vi "Control Panel.vi"(8 "error in (no error)":errorcluster, 11 "Lockin SR830.lvclass":refnum<class "Lockin SR830.lvclass">) -> (0 "error out":errorcluster, 3 "Lockin SR830.lvclass out":refnum<class "Lockin SR830.lvclass">)   [LabVIEW 2009, in "Lockin SR830.lvclass"]
uses:
  Lockin SR830.lvclass
  sr830/SR830.lvlib
  Main/Global/Misc.vi
  Main/Global/Flags.vi
  Global/GPIB Numbers.vi
  Utility Classes/Readable/Readable.lvclass
panel:
  out "ext?OUT":bool
  in  "ext?":bool caption="External Lock"
  in  "ch2form":T1(ring)
  in  "readcontrol":bool
  in  "ch1form":enum16{"X", "R", "X Noise", "Aux 1", "Aux 2"}(ring)
  in  "reset":bool
  out "frequnit":string
  out "freq":dbl caption="Ref Freq"
  out "ch2format":string
  out "ch1format":string
  out "ch2disp":string caption="Channel 2"
  out "ch1disp":string caption="Channel 1"
  in  "readtime":dbl=500.0 caption="Read Time (ms)"
  in  "activeread":bool caption="Auto-read?"
  in  "autophase":bool
  out "phasedisp":dbl caption="Phase"
  out "on":bool caption="Connected"
  out "sensdisp":T2(ring) caption="Sensitivity"
  out "tcdisp":T3(ring) caption="Time Const."
  in  "sens":T2(ring) caption="Sensitivity"
  in  "tc":T3(ring) caption="Time Const."
  in  "connect":bool
  in  "set":bool
  in  "read":bool
  out "active":bool caption="Active"
  in  "endprgm":bool
  # "Lock-in Detector Front Panel"
  # "**Auto-read is just for the output data."
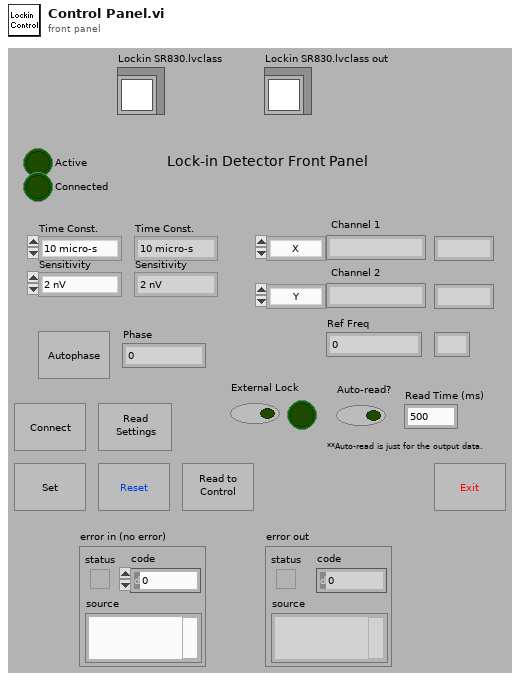
[diagram p1: front panel]
types:
  T1 = enum16{"Y", "Theta", "Y Noise", "Aux 3", "Aux 4"}
  T2 = enum16{"2 nV", "5 nV", "10 nV", "20 nV", "50 nV", "100 nV", "200 nV", "500 nV", "1 microV", "2 microV", "5 microV", "10 microV", "20 microV", "50  microV", "100  microV", "200  microV", "500  microV", "1 mV", "2 mV", "5 mV", "10 mV", "20 mV", "50 mV", "100 mV", "200  mV", "500 mV", "1 V"}
  T3 = enum16{"10 micro-s", "30 micro-s", "100 micro-s", "300 micro-s", "1 ms", "3 ms", "10 ms", "30 ms", "100 ms", "300 ms", "1 s", "3 s", "10 s", "30 s", "100 s", "300 s", "1000 s", "30000 s", "10 ks", "30 ks"}
  T4 = cluster{"name":string, "value":dbl, "unit":string}[]
  T5 = typedef "GPIB Type Def.ctl" = cluster{"Name":string, "bus":dbl, "GPIB":dbl, "GPIB as string":string, "byte":i32, "VISA Resource Name":refnum<visa-resource-name>}
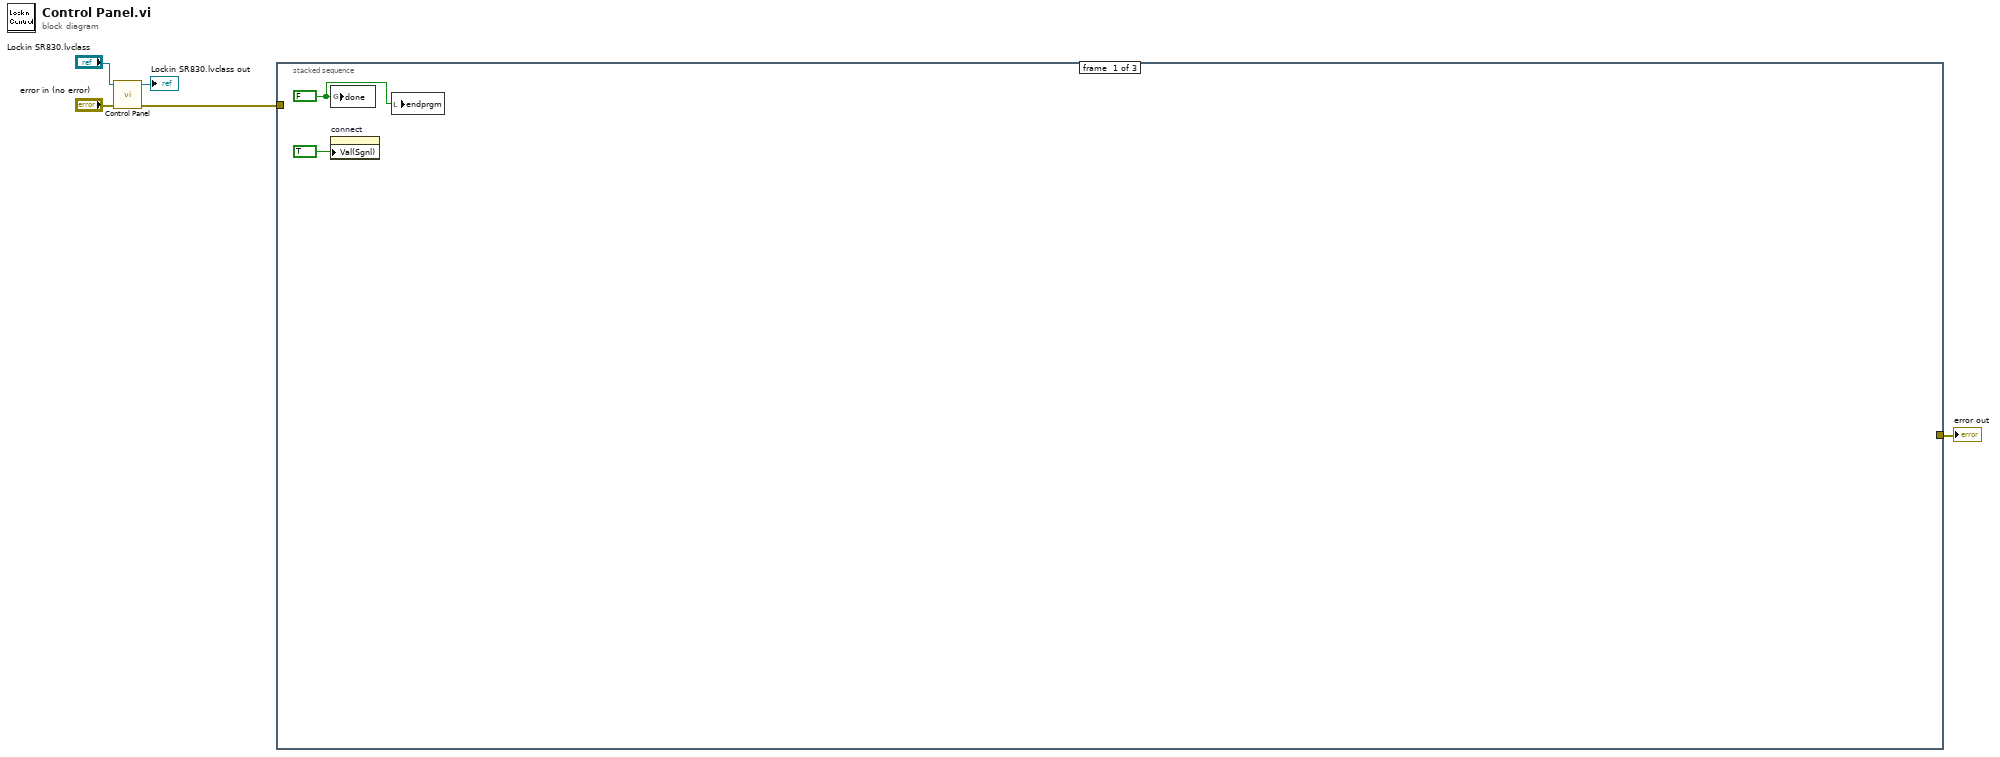
[diagram p0: block diagram]
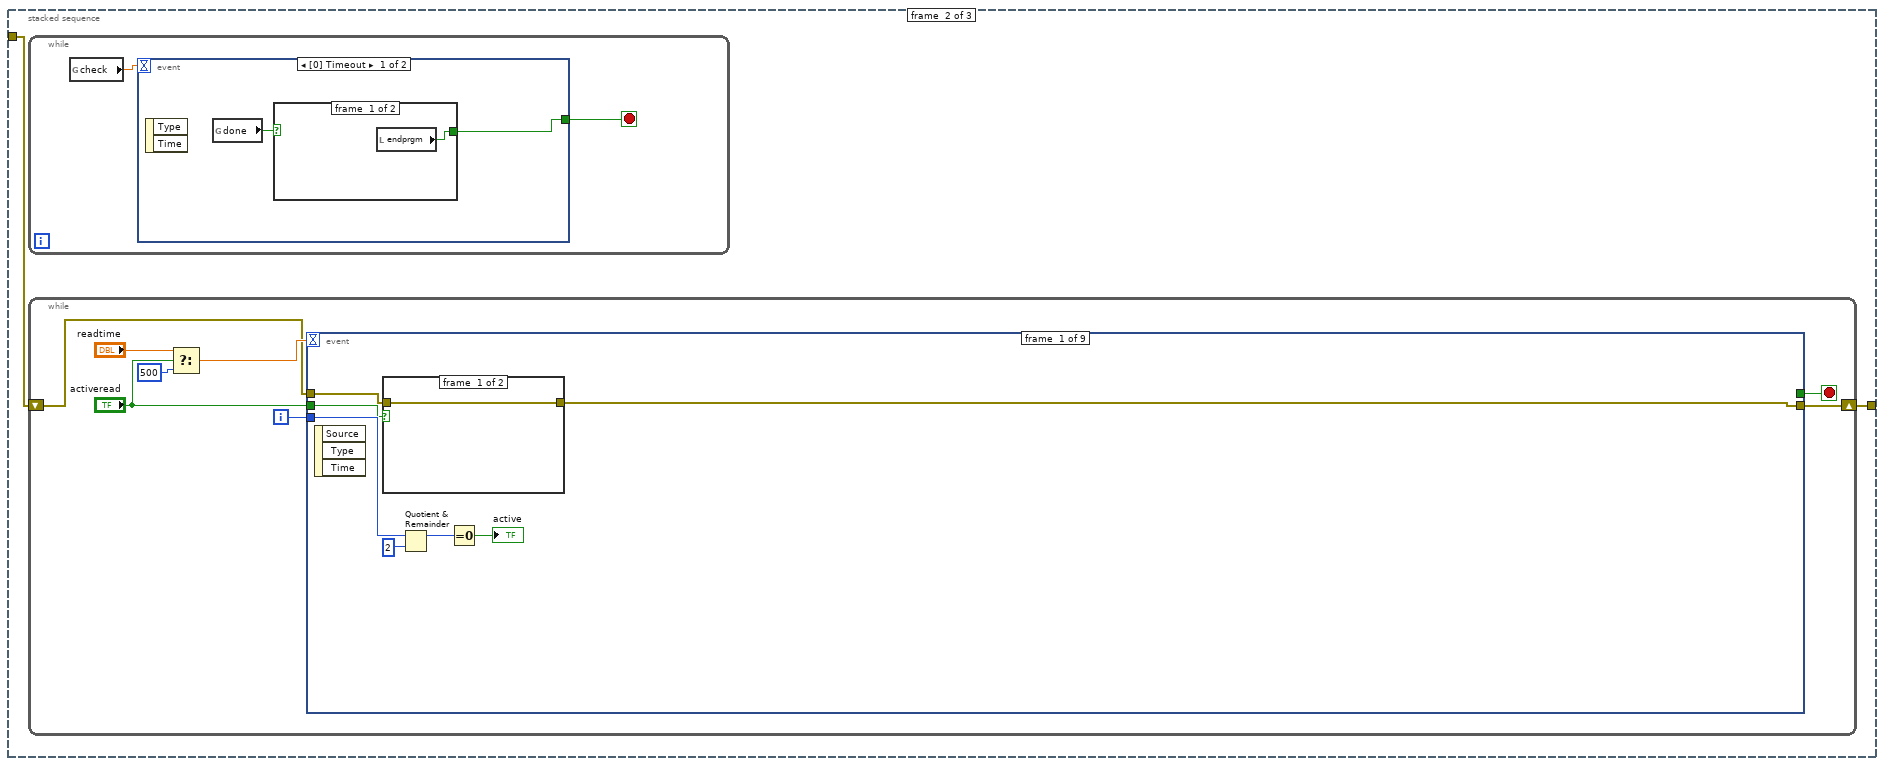
[diagram p2: hidden frame]
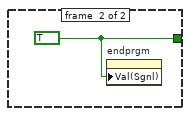
[diagram p3: hidden frame]
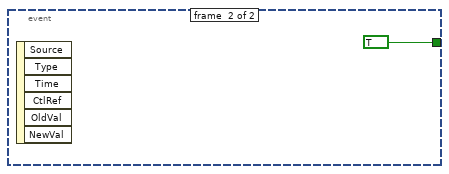
[diagram p4: hidden frame]
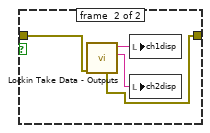
[diagram p5: hidden frame]
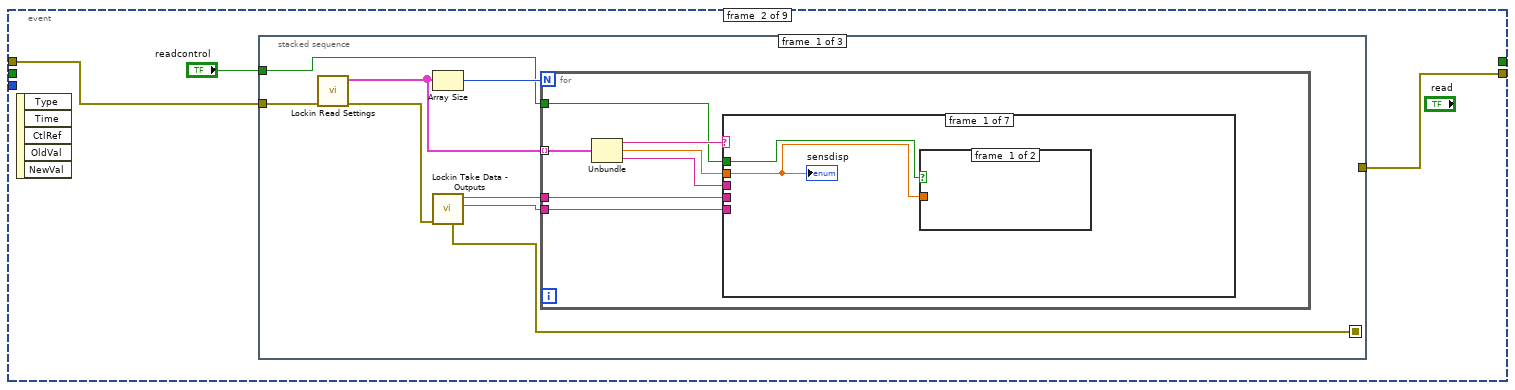
[diagram p6: hidden frame]
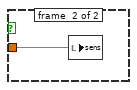
[diagram p7: hidden frame]
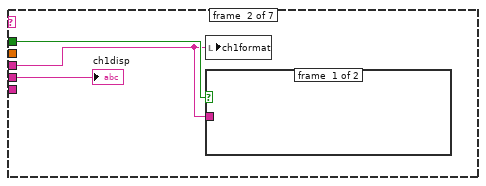
[diagram p8: hidden frame]
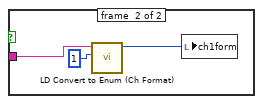
[diagram p9: hidden frame]
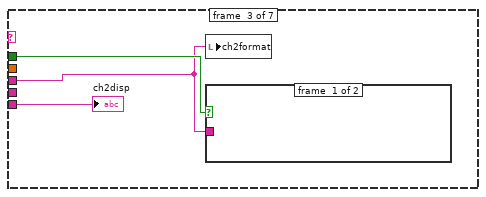
[diagram p10: hidden frame]
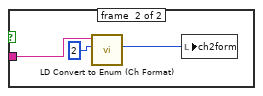
[diagram p11: hidden frame]
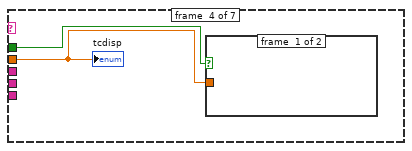
[diagram p12: hidden frame]
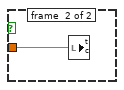
[diagram p13: hidden frame]
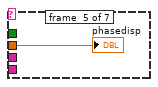
[diagram p14: hidden frame]
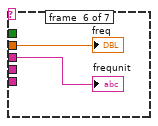
[diagram p15: hidden frame]
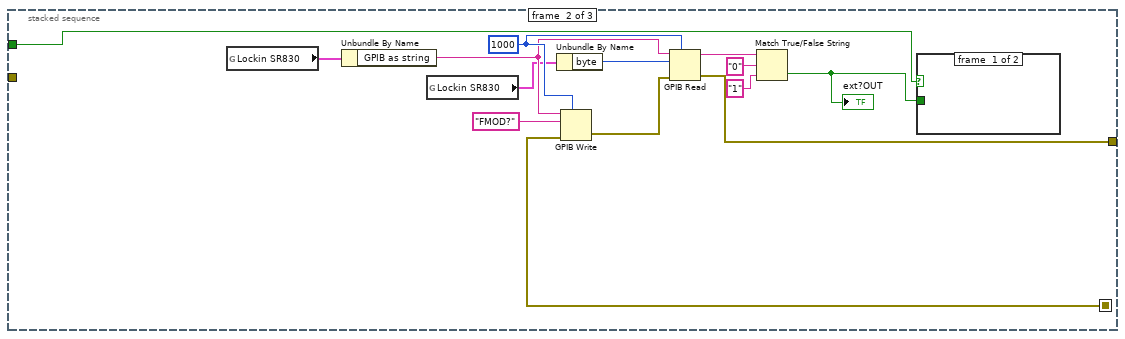
[diagram p17: hidden frame]
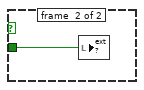
[diagram p18: hidden frame]
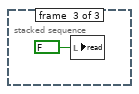
[diagram p19: hidden frame]
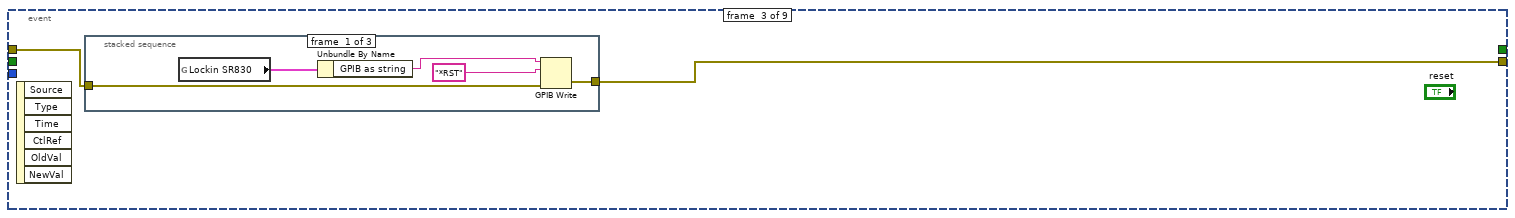
[diagram p20: hidden frame]
diagram:
  n1 = call-parent "Control Panel.vi"("error in (no error)"="error in (no error)", "Instrument in"="Lockin SR830.lvclass") -> ("error out"=w3:errorcluster, "Instrument out"=→"Lockin SR830.lvclass out":refnum<class "Lockin SR830.lvclass">)  [unwired: 8 in]
  n2 = stacked-sequence {
    tunnel: w3 -> [_ w9 _]
    tunnel: [_ w8 _] -> w1
    frame #0 {
      w7 = FALSE
      n3 = global write "Flags.vi" "done"(w7) -> ()
      n4 = property on="connect" class="Bool (strict)"("Val(Sgnl)"=TRUE) -> ()  [unwired: 2 in, 2 out]
      n5 = local write "endprgm"(w7) -> ()
    }
    frame #1 {
      n6 = while {
        stop <- w11 stop-if-true
        n7 = global read "Misc.vi" "check"() -> (w10:dbl)
        n8 = event shown="[0] Timeout" {
          selector: _ -> [_ _]
          dyn-events: _ -> [_ _]
          timeout: w10 -> [_ _]
          tunnel: [w12 TRUE] -> w11
          event #0 {
            n9 = event-data() -> ()  [unwired: 3 out]
            n10 = global read "Flags.vi" "done"() -> (w13:bool)
            n11 = case shown="False" w13 {
              tunnel: [w14 w15] -> w12
              frame #0 {
                n12 = local read "endprgm"() -> (w14:bool)
              }
              frame #1 {
                w15 = TRUE
                n13 = property on="endprgm" class="Bool (strict)"("Val(Sgnl)"=w15) -> ()  [unwired: 2 in, 2 out]
              }
            }
          }
          event #1 {
            n14 = event-data() -> ()  [unwired: 7 out]
          }
        }
      }
      n15 = while {
        shift-right: [w18] -> w8
        shift-left: w9 -> [w19]
        i -> [w23]
        stop <- w24 stop-if-true
        n16 = Select(t="readtime", s="activeread", f=500) -> (s? t:f=w20:dbl)
        n17 = event shown="[4] \"set\": Value Change" {
          selector: _ -> [_ _ _ _ _ _ _ _ _]
          dyn-events: _ -> [_ _ _ _ _ _ _ _ _]
          timeout: w20 -> [_ _ _ _ _ _ _ _ _]
          tunnel: [_ _ _ _ _ _ _ _ "endprgm"] -> w24
          tunnel: w23 -> [w28 _ _ _ _ _ _ _ _]
          tunnel: w19 -> [w26 w39 w93 _ w159 w193 w203 w220 w221]
          tunnel: [w25 w38 w92 w100 w158 w189 w202 w220 w221] -> w18
          tunnel: "activeread" -> [w27 _ _ _ _ _ _ _ _]
          event #0 {
            n18 = event-data() -> ()  [unwired: 4 out]
            n19 = case shown="True" w27 {
              tunnel: w26 -> [w32 w36]
              tunnel: [w32 w35] -> w25
              frame #0 {
              }
              frame #1 {
                n20 = call "Lockin Take Data - Outputs.vi"("error in (no error)"=w36) -> ("output2"=w33:string, "output1"=w34:string, "error out"=w35:errorcluster)  [unwired: 8 out]
                n21 = local write "ch1disp"(w34) -> ()
                n22 = local write "ch2disp"(w33) -> ()
              }
            }
            n23 = Quotient & Remainder(x=w28, y=2) -> (x-y*floor(x/y)=w30:i32)  [unwired: 1 out]
            n24 = Equal To 0?(x=w30) -> (x = 0?=→"active":bool)
          }
          event #1 {
            n25 = event-data() -> ()  [unwired: 6 out]
            n26 = stacked-sequence {
              seq-local: [w41 _ _] -> [_ w82 _]
              tunnel: w39 -> [w43 _ _]
              tunnel: [_ w81 _] -> w38
              tunnel: "readcontrol" -> [w40 w77 _]
              frame #0 {
                n27 = call "Lockin Read Settings.vi"("errorIN"=w43) -> ("errorOUT"=w42:errorcluster, "lockinsettings"=w46:T4)  [unwired: 9 out]
                n28 = Array Size(array=w46) -> (size(s)=w47:i32)
                n29 = call "Lockin Take Data - Outputs.vi"("error in (no error)"=w42) -> ("output2"=w44:string, "output1"=w45:string, "error out"=w41:errorcluster)  [unwired: 8 out]
                n30 = for {
                  N: w47 -> [_]
                  tunnel: w46 -> [w54] mode=indexing
                  tunnel: w45 -> [w52]
                  tunnel: w44 -> [w51]
                  tunnel: w40 -> [w48]
                  n31 = Unbundle(w54) -> ("name"=w53:string, "value"=w50:dbl, "unit"=w49:string)
                  n32 = case shown="\"LDch2disp\"" w53 {
                    tunnel: w52 -> [_ w59 _ _ _ _ _]
                    tunnel: w51 -> [_ _ w66 _ _ _ _]
                    tunnel: w50 -> [w55 _ _ w70 w73 w74 _]
                    tunnel: w49 -> [_ w58 w64 _ _ w75 _]
                    tunnel: w48 -> [w56 w60 w65 w71 _ _ _]
                    frame #0 {
                      n33 = case shown="True" w56 {
                        tunnel: w55 -> [_ w57]
                        frame #0 {
                        }
                        frame #1 {
                          n34 = local write "sens"(w57) -> ()
                        }
                      }
                      "sensdisp" <- w55
                    }
                    frame #1 {
                      n35 = local write "ch1format"(w58) -> ()
                      n36 = case shown="True" w60 {
                        tunnel: w58 -> [_ w63]
                        frame #0 {
                        }
                        frame #1 {
                          n37 = call "LD Convert to Enum (Ch Format).vi"("channel"=1, "stringIN"=w63) -> ("ch1form"=w61:enum16{"X", "R", "X Noise", "Aux 1", "Aux 2"})  [unwired: 9 out]
                          n38 = local write "ch1form"(w61) -> ()
                        }
                      }
                      "ch1disp" <- w59
                    }
                    frame #2 {
                      n39 = local write "ch2format"(w64) -> ()
                      n40 = case shown="True" w65 {
                        tunnel: w64 -> [_ w69]
                        frame #0 {
                        }
                        frame #1 {
                          n41 = call "LD Convert to Enum (Ch Format).vi"("channel"=2, "stringIN"=w69) -> ("ch2form"=w67:T1)  [unwired: 9 out]
                          n42 = local write "ch2form"(w67) -> ()
                        }
                      }
                      "ch2disp" <- w66
                    }
                    frame #3 {
                      n43 = case shown="True" w71 {
                        tunnel: w70 -> [_ w72]
                        frame #0 {
                        }
                        frame #1 {
                          n44 = local write "tc"(w72) -> ()
                        }
                      }
                      "tcdisp" <- w70
                    }
                    frame #4 {
                      "phasedisp" <- w73
                    }
                    frame #5 {
                      "freq" <- w74
                      "frequnit" <- w75
                    }
                    frame #6 {
                    }
                  }
                }
              }
              frame #1 {
                w89 = 1000
                n45 = global read "GPIB Numbers.vi" "Lockin SR830"() -> (w84:T5)
                n46 = Unbundle By Name(w84) -> ("GPIB as string"=w88:string)
                n47 = global read "GPIB Numbers.vi" "Lockin SR830"() -> (w86:T5)
                n48 = Unbundle By Name(w86) -> ("byte"=w87:i32)
                n49 = GPIB Write(0:w88, 1:"FMOD?", 3:w82, 4:w89) -> (6:w85:errorcluster)  [unwired: 2 out]
                n50 = GPIB Read(0:w88, 1:w87, 3:w85, 4:w89) -> (5:w80:string, 7:w81:errorcluster)  [unwired: 2 out]
                n51 = Match True/False String(2:"1", 3:"0", 4:w80) -> (0:w76:bool)  [unwired: 1 out]
                "ext?OUT" <- w76
                n52 = case shown="True" w77 {
                  tunnel: w76 -> [_ w90]
                  frame #0 {
                  }
                  frame #1 {
                    n53 = local write "ext?"(w90) -> ()
                  }
                }
              }
              frame #2 {
                n54 = local write "read"(FALSE) -> ()
              }
            }
          }
          event #2 {
            n55 = event-data() -> ()  [unwired: 7 out]
            n56 = stacked-sequence {
              tunnel: w93 -> [w95 _ _]
              tunnel: [w94 _ _] -> w92
              frame #0 {
                n57 = global read "GPIB Numbers.vi" "Lockin SR830"() -> (w98:T5)
                n58 = Unbundle By Name(w98) -> ("GPIB as string"=w97:string)
                n59 = GPIB Write(0:w97, 1:"*RST", 3:w95) -> (6:w94:errorcluster)  [unwired: 3 out]
              }
              frame #1 {
                n60 = Wait (ms)(milliseconds to wait=150) -> ()  [unwired: 1 out]
              }
              frame #2 {
              }
            }
          }
          event #3 {
            n61 = event-data() -> ()  [unwired: 2 out]
            n62 = local write "connect"(FALSE) -> ()
            n63 = call "Lockin Initialize.vi"() -> ("errorOUT"=w101:errorcluster, "ready?"=w103:bool)  [unwired: 1 in, 9 out]
            "on" <- w103
            n64 = case shown="True" w103 {
              tunnel: w101 -> [w104 w117]
              tunnel: [w104 w109] -> w100
              frame #0 {
              }
              frame #1 {
                n65 = call "Lockin Read Settings.vi"("errorIN"=w117) -> ("errorOUT"=w116:errorcluster, "lockinsettings"=w120:T4)  [unwired: 9 out]
                n66 = call "Lockin Take Data - Outputs.vi"("error in (no error)"=w116) -> ("output2"=w118:string, "output1"=w119:string, "error out"=w110:errorcluster)  [unwired: 8 out]
                n67 = global read "GPIB Numbers.vi" "Lockin SR830"() -> (w115:T5)
                n68 = for {
                  tunnel: w120 -> [w126] mode=indexing
                  tunnel: w119 -> [w124]
                  tunnel: w118 -> [w123]
                  n69 = Unbundle(w126) -> ("name"=w125:string, "value"=w122:dbl, "unit"=w121:string)
                  n70 = case shown="\"LDch2disp\"" w125 {
                    tunnel: w124 -> [_ w129 _ _ _ _ _]
                    tunnel: w123 -> [_ _ w131 _ _ _ _]
                    tunnel: w122 -> [w127 _ _ w132 w133 w134 _]
                    tunnel: w121 -> [_ w128 w130 _ _ w135 _]
                    frame #0 {
                      n71 = local write "sensdisp"(w127) -> ()
                    }
                    frame #1 {
                      n72 = local write "ch1disp"(w129) -> ()
                      n73 = local write "ch1format"(w128) -> ()
                    }
                    frame #2 {
                      n74 = local write "ch2disp"(w131) -> ()
                      n75 = local write "ch2format"(w130) -> ()
                    }
                    frame #3 {
                      n76 = local write "tcdisp"(w132) -> ()
                    }
                    frame #4 {
                      n77 = local write "phasedisp"(w133) -> ()
                    }
                    frame #5 {
                      n78 = local write "freq"(w134) -> ()
                      n79 = local write "frequnit"(w135) -> ()
                    }
                    frame #6 {
                    }
                  }
                }
                n80 = Unbundle By Name(w115) -> ("GPIB as string"=w114:string, "byte"=w111:i32)
                n81 = GPIB Write(0:w114, 1:"FMOD?", 3:w110) -> (6:w112:errorcluster)  [unwired: 3 out]
                n82 = GPIB Read(0:w114, 1:w111, 3:w112) -> (5:w108:string, 7:w109:errorcluster)  [unwired: 3 out]
                n83 = Match True/False String(2:"1", 3:"0", 4:w108) -> (0:w105:bool)  [unwired: 1 out]
                n84 = local write "ext?OUT"(w105) -> ()
              }
            }
          }
          event #4 {
            n85 = event-data() -> ()  [unwired: 7 out]
            n86 = To Long Integer(number="tc") -> (32bit integer=w168:i32)
            n87 = To Long Integer(number="sens") -> (32bit integer=w167:i32)
            n88 = Number To Decimal String(number=w168) -> (decimal integer string=w165:string)  [unwired: 1 out]
            n89 = global read "GPIB Numbers.vi" "Lockin SR830"() -> (w171:T5)
            n90 = Number To Decimal String(number="ch1form") -> (decimal integer string=w151:string)  [unwired: 1 out]
            n91 = Number To Decimal String(number=w167) -> (decimal integer string=w163:string)  [unwired: 1 out]
            n92 = Concatenate Strings("OFLT ", w165) -> (w164:string)
            n93 = Unbundle By Name(w171) -> ("GPIB as string"=w144:string)
            n94 = local read "ext?"() -> (w138:bool)
            n95 = Number To Decimal String(number="ch2form") -> (decimal integer string=w149:string)  [unwired: 1 out]
            n96 = Concatenate Strings("SENS ", w163) -> (w161:string)
            n97 = Not(x=w138) -> (.not. x?=w137:bool)
            n98 = GPIB Write(0:w144, 1:w164, 3:w159) -> (6:w160:errorcluster)  [unwired: 3 out]
            n99 = Boolean To (0,1)(Boolean=w137) -> (0, 1=w136:i16)
            n100 = Concatenate Strings("DDEF 1, ", w151, ",0") -> (w148:string)
            n101 = Number To Decimal String(number=w136) -> (decimal integer string=w140:string)  [unwired: 1 out]
            n102 = GPIB Write(0:w144, 1:w161, 3:w160) -> (6:w156:errorcluster)  [unwired: 3 out]
            n103 = Concatenate Strings("DDEF 2, ", w149, ",0") -> (w147:string)
            n104 = GPIB Write(0:w144, 1:w148, 3:w156) -> (6:w155:errorcluster)  [unwired: 3 out]
            n105 = Concatenate Strings("FMOD ", w140) -> (w139:string)
            n106 = GPIB Write(0:w144, 1:w147, 3:w155) -> (6:w143:errorcluster)  [unwired: 3 out]
            n107 = GPIB Write(0:w144, 1:w139, 3:w143) -> (6:w142:errorcluster)  [unwired: 1 in, 2 out]
            n108 = call "Lockin Read Settings.vi"("errorIN"=w142) -> ("errorOUT"=w158:errorcluster, "lockinsettings"=w157:T4)  [unwired: 9 out]
            n109 = for {
              tunnel: w157 -> [w175] mode=indexing
              n110 = Unbundle(w175) -> ("name"=w174:string, "value"=w173:dbl, "unit"=w172:string)
              n111 = case shown="\"LDch1disp\"" w174 {
                tunnel: w173 -> [_ w176 w177 _ _ w181]
                tunnel: w172 -> [_ _ _ w178 w179 w180]
                frame #0 {
                }
                frame #1 {
                  n112 = local write "sensdisp"(w176) -> ()
                }
                frame #2 {
                  n113 = local write "tcdisp"(w177) -> ()
                }
                frame #3 {
                  "ch1format" <- w178
                }
                frame #4 {
                  "ch2format" <- w179
                }
                frame #5 {
                  n114 = local write "freq"(w181) -> ()
                  n115 = local write "frequnit"(w180) -> ()
                }
              }
            }
          }
          event #5 {
            n116 = event-data() -> ()  [unwired: 7 out]
            n117 = Not(x="ext?") -> (.not. x?=w197:bool)
            n118 = Boolean To (0,1)(Boolean=w197) -> (0, 1=w198:i16)
            n119 = Number To Decimal String(number=w198) -> (decimal integer string=w196:string)  [unwired: 1 out]
            n120 = global read "GPIB Numbers.vi" "Lockin SR830"() -> (w194:T5)
            n121 = Unbundle By Name(w194) -> ("byte"=w187:i32, "GPIB as string"=w188:string)
            n122 = Concatenate Strings("FMOD ", w196) -> (w199:string)
            n123 = GPIB Write(0:w188, 1:w199, 3:w193) -> (6:w191:errorcluster)  [unwired: 1 in, 2 out]
            n124 = GPIB Write(0:w188, 1:"FMOD?", 3:w191) -> (6:w190:errorcluster)  [unwired: 1 in, 2 out]
            n125 = GPIB Read(0:w188, 1:w187, 3:w190) -> (5:w184:string, 7:w189:errorcluster)  [unwired: 1 in, 2 out]
            n126 = Match True/False String(2:"1", 3:"0", 4:w184) -> (0:w182:bool)  [unwired: 1 out]
            n127 = local write "ext?OUT"(w182) -> ()
          }
          event #6 {
            n128 = event-data() -> ()  [unwired: 7 out]
            n129 = global read "GPIB Numbers.vi" "Lockin SR830"() -> (w201:T5)
            n130 = Unbundle By Name(w201) -> ("GPIB as string"=w200:string)
            n131 = stacked-sequence {
              seq-local: [w204 _ _] -> [_ _ w209]
              tunnel: w203 -> [w206 _ _]
              tunnel: [_ _ w210] -> w202
              tunnel: w200 -> [w205 _ w218]
              frame #0 {
                n132 = GPIB Write(0:w205, 1:"APHS", 3:w206) -> (6:w204:errorcluster)  [unwired: 3 out]
              }
              frame #1 {
                n133 = Wait (ms)(milliseconds to wait=50) -> ()  [unwired: 1 out]
              }
              frame #2 {
                n134 = global read "GPIB Numbers.vi" "Lockin SR830"() -> (w216:T5)
                n135 = Unbundle By Name(w216) -> ("byte"=w215:i32)
                n136 = GPIB Write(0:w218, 1:"PHAS?", 3:w209) -> (6:w219:errorcluster)  [unwired: 3 out]
                n137 = GPIB Read(0:w218, 1:w215, 2:2, 3:w219) -> (5:w212:string, 7:w213:errorcluster)  [unwired: 2 out]
                n138 = Scan From String(input string=w212, error in=w213) -> (error out=w210:errorcluster, output 1=w211:dbl)  [unwired: 2 in, 3 out]
                n139 = local write "phasedisp"(w211) -> ()
              }
            }
          }
          event #7 {
            n140 = event-data() -> ()  [unwired: 7 out]
          }
          event #8 {
            n141 = event-data() -> ()  [unwired: 7 out]
          }
        }
      }
    }
    frame #2 {
      n142 = local write "endprgm"(FALSE) -> ()
    }
  }
  "error out" <- w1
